vi "onJobCancelled.vi"(8 "error in (no error)":errorcluster, 11 "Job in":refnum<class "Job.lvclass">) -> (0 "error out":errorcluster, 3 "Job out":refnum<class "Job.lvclass">)   [LabVIEW 2013, in "openCron.lvlib" / "Job.lvclass"]
uses:
  Job.lvclass
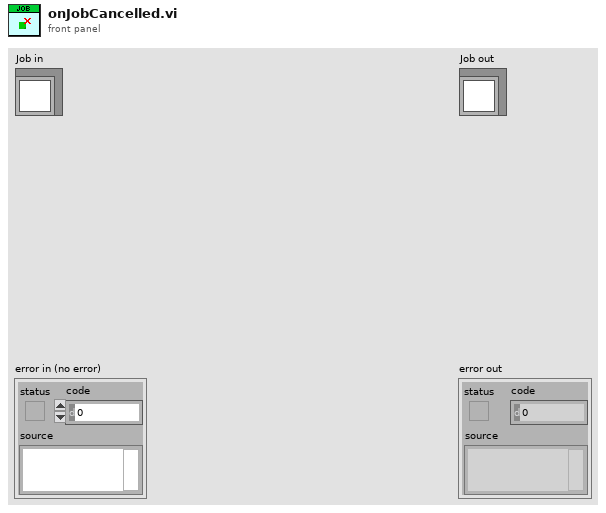
[diagram p1: front panel]
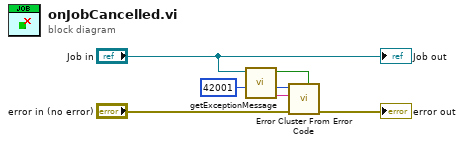
[diagram p0: block diagram]
diagram:
  n1 = call-dynamic "getExceptionMessage.vi"("exception"=42001, "Job in"="Job in") -> ("exception message"=w6:string, "exception dup"=w7:i32, "warning?"=w5:bool)  [unwired: 7 in]
  n2 = call <vilib>:"Error Cluster From Error Code.vi"("is warning? (False)"=w5, "error in (no error)"="error in (no error)", "error message (\"\")"=w6, "error code (0)"=w7) -> ("error out"=→"error out":errorcluster)  [unwired: 5 in]
  "Job out" <- "Job in"
